vi "MotionMagicDutyCycle SetControl.vi"(0 "DeviceReference":T1, 1 "Position":dbl, 2 "EnableFOC":bool=TRUE, 3 "FeedForward":dbl, 4 "Slot":i32, 5 "OverrideBrakeDurNeutral":bool, 6 "LimitForwardMotion":bool, 7 "error in":errorcluster, 8 "LimitReverseMotion":bool, 9 "IgnoreHardwareLimits":bool, 10 "UseTimesync":bool, 18 "Update Frequency (Hz)":dbl=100.0) -> (20 "DeviceReference Out":T1, 27 "error out":errorcluster)   [LabVIEW 2023]
doc: "Requests Motion Magic® to target a final position using a motion profile. Users can optionally provide a duty cycle feedforward.\nMotion Magic® produces a motion profile in real-time while attempting to honor the Cruise Velocity, Acceleration, and (optional) Jerk specified via the Motion Magic® configuration values. This control mode does not use the Expo_kV or Expo_kA configs.\nTarget position can be changed on-the-fly and Motion Magic® will do its best to adjust the profile. This control mode is duty cycle based, so relevant closed-loop gains will use fractional duty cycle for the numerator: +1.0 represents full forward output."
uses:
  <vilib>/Rock Robotics/WPI/ThirdParty/Phoenix6/DeviceReference.ctl
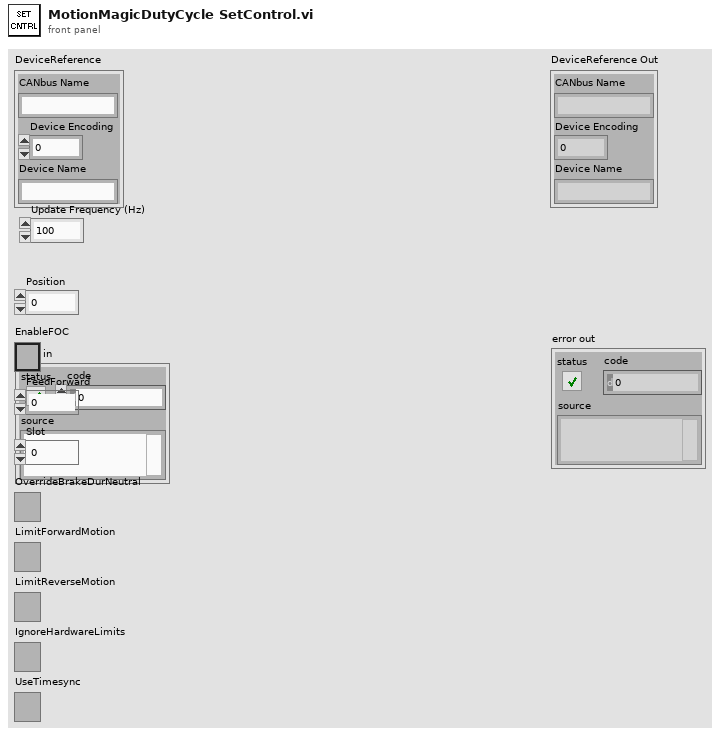
[diagram p1: front panel]
types:
  T1 = typedef "DeviceReference.ctl" = cluster{"CANbus Name":string, "Device Encoding":u32, "Device Name":string}
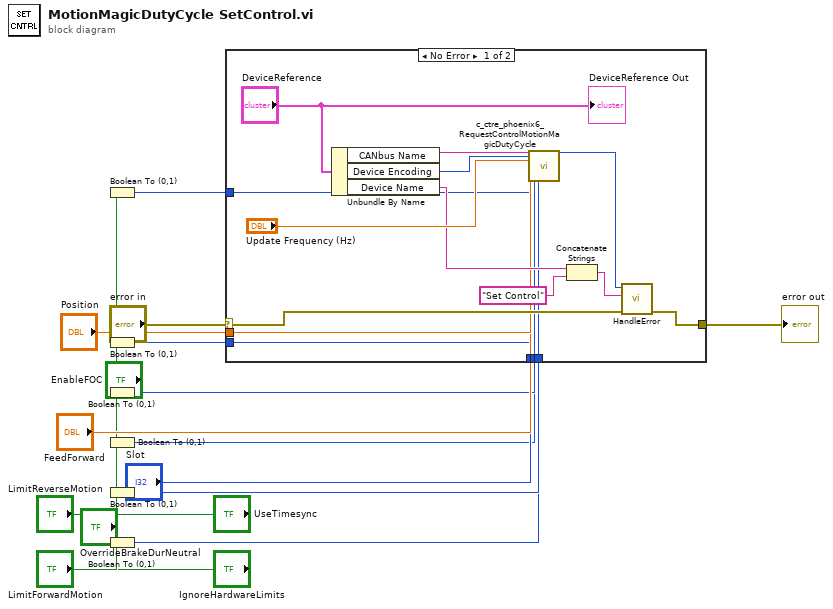
[diagram p0: block diagram]
diagram:
  n1 = Boolean To (0,1)(Boolean="EnableFOC") -> (0, 1=w13:i16)
  n2 = Boolean To (0,1)(Boolean="OverrideBrakeDurNeutral") -> (0, 1=w9:i16)
  n3 = Boolean To (0,1)(Boolean="LimitForwardMotion") -> (0, 1=w7:i16)
  n4 = Boolean To (0,1)(Boolean="LimitReverseMotion") -> (0, 1=w5:i16)
  n5 = Boolean To (0,1)(Boolean="IgnoreHardwareLimits") -> (0, 1=w3:i16)
  n6 = Boolean To (0,1)(Boolean="UseTimesync") -> (0, 1=w1:i16)
  n7 = case shown="No Error" "error in" {
    selector: "error in" -> [w31 w37]
    tunnel: [w30 w37] -> w16
    tunnel: "Position" -> [w26 _]
    tunnel: w13 -> [w25 _]
    tunnel: "FeedForward" -> [w24 _]
    tunnel: "Slot" -> [w23 _]
    tunnel: w9 -> [w22 _]
    tunnel: w7 -> [w21 _]
    tunnel: w5 -> [w20 _]
    tunnel: w3 -> [w19 _]
    tunnel: w1 -> [w18 _]
    frame No Error {
      n8 = Unbundle By Name("DeviceReference") -> ("CANbus Name"=w35:string, "Device Encoding"=w34:u32, "Device Name"=w29:string)
      n9 = call <vilib>:"c_ctre_phoenix6_RequestControlMotionMagicDutyCycle.vi"("String 2"=w35, "Numeric 2"=w34, "Numeric 3"="Update Frequency (Hz)", "Numeric 4"=w26, "Numeric 5"=w25, "Numeric 6"=w24, "Numeric 7"=w23, "Numeric 8"=w22, "Numeric 9"=w21, "Numeric 10"=w20, "Numeric 11"=w19, "Numeric 12"=w18) -> ("Numeric"=w32:i32)  [unwired: 14 in, 1 out]
      n10 = Concatenate Strings(w29, "Set Control" ("origin")) -> (w27:string)
      n11 = call <vilib>:"HandleError.vi"("error in"=w31, "origin"=w27, "Status"=w32) -> ("error out"=w30:errorcluster)  [unwired: 8 in]
      "DeviceReference Out" <- "DeviceReference"
    }
    frame Error {
    }
  }
  "error out" <- w16
